vi "test.vi"() -> ()   [LabVIEW 2016, in "ProgrammaticInitialization.lvclass"]
uses:
  ProgrammaticInitialization.lvclass
panel:
  out "error out":errorcluster
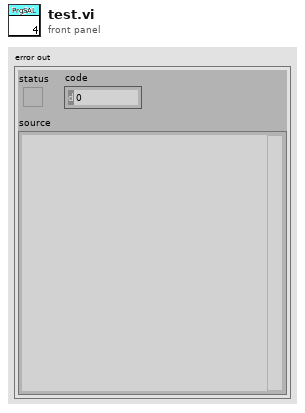
[diagram p1: front panel]
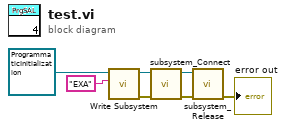
[diagram p0: block diagram]
diagram:
  n1 = call-dynamic "Write Subsystem.vi"("Subsystem"="EXA", "ProgrammaticInitialization in"=refnum<class "ProgrammaticInitialization.lvclass"> refnum) -> ("error out"=w2:errorcluster, "ProgrammaticInitialization out"=w5:refnum<class "ProgrammaticInitialization.lvclass">)  [unwired: 8 in]
  n2 = call "subsystem_Connect.vi"("error in (no error)"=w2, "ProgrammaticInitialization in"=w5) -> ("error out"=w7:errorcluster, "ProgrammaticInitialization out"=w1:refnum<class "ProgrammaticInitialization.lvclass">)  [unwired: 8 in]
  n3 = call "subsystem_Release.vi"("error in (no error)"=w7, "ProgrammaticInitialization in"=w1) -> ("error out"=→"error out":errorcluster)  [unwired: 8 in, 1 out]
